vi "ABB configure locked rotor.vi"() -> ()   [LabVIEW 2017]
uses:
  ABB global.vi
panel:
  in  "Exit":bool
  in  "Locked Rotor Test":T1={"Number Values"=8, "Tolerance (%)"=2.0, "Value (% rated) "=[1.15, 1.0, 0.91, 0.78, 0.66, 0.55, 0.42, 0.3], "Hold time (sec)"=2.0}
  # "Configure Locked Rotor Test"
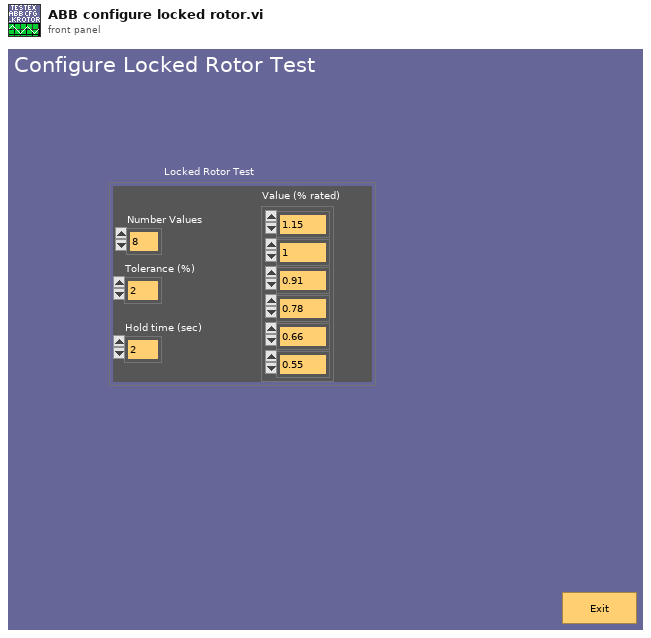
[diagram p1: front panel]
types:
  T1 = cluster{"Number Values":i32, "Tolerance (%)":dbl, "Value (% rated) ":dbl[], "Hold time (sec)":dbl}
  T2 = cluster{"Number Values":i32, "Tolerance":dbl, "Value (ratio) ":dbl[], "Hold time (sec)":dbl}
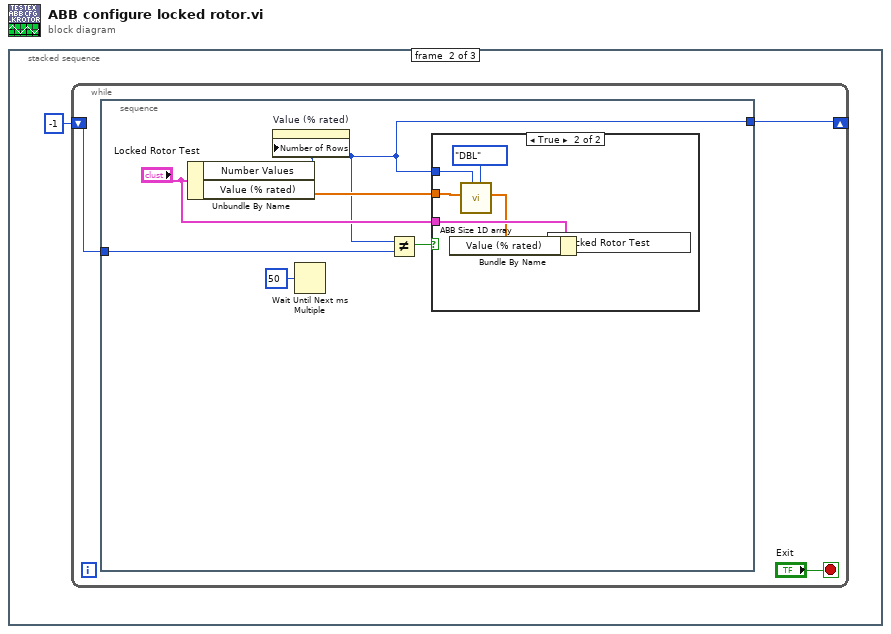
[diagram p0: block diagram]
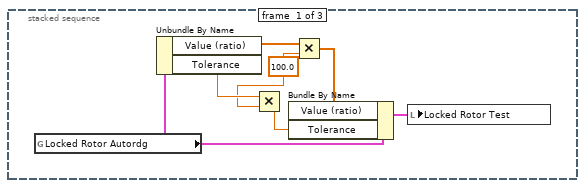
[diagram p2: hidden frame]
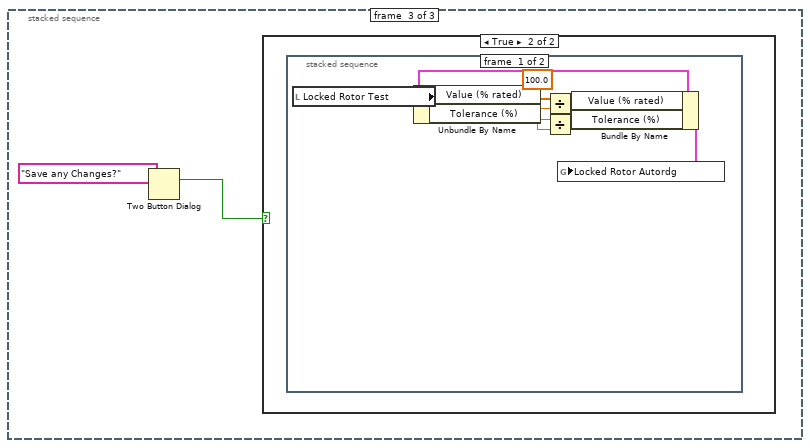
[diagram p4: hidden frame]
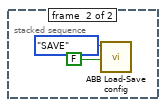
[diagram p6: hidden frame]
diagram:
  n1 = stacked-sequence {
    frame #0 {
      w2 = 100.0
      n2 = global read "ABB global.vi" "Locked Rotor Autordg"() -> (w6:T2)
      n3 = Unbundle By Name(w6) -> ("Value (ratio)"=w7:dbl[], "Tolerance"=w3:dbl)
      n4 = Multiply(x=w3, y=w2) -> (x*y=w1:dbl)
      n5 = Multiply(x=w7, y=w2) -> (x*y=w5:dbl[])
      n6 = Bundle By Name(cluster=w6, "Value (ratio)"=w5, "Tolerance"=w1) -> (w4:T2)
      n7 = local write "Locked Rotor Test"(w4) -> ()
    }
    frame #1 {
      n8 = while {
        shift-right: [w9] -> _
        shift-left: -1 ("Number Values") -> [w10]
        stop <- "Exit" stop-if-true
        n9 = stacked-sequence {
          tunnel: w10 -> [w15]
          tunnel: [w12] -> w9
          frame #0 {
            n10 = Unbundle By Name("Locked Rotor Test") -> ("Number Values"=w12:i32, "Value (% rated)"=w13:dbl[])
            n11 = property on="Value (% rated)" class="Arr (strict)"("Number of Rows"=w12) -> ()  [unwired: 2 in, 2 out]
            n12 = Wait Until Next ms Multiple(millisecond multiple=u32 50) -> ()  [unwired: 1 out]
            n13 = Not Equal?(x=w12, y=w15) -> (x != y?=w14:bool)
            n14 = case shown="True" w14 {
              tunnel: "Locked Rotor Test" -> [_ w23]
              tunnel: w13 -> [_ w21]
              tunnel: w12 -> [_ w19]
              frame False {
              }
              frame True {
                n15 = call "ABB Size 1D array.vi"("Type"=enum16{"Integer", "DBL", "STRING", "BOOLEAN"}."DBL", "Size"=w19, "DBL Array In"=w21) -> ("DBL Array out"=w18:dbl[])  [unwired: 5 in, 3 out]
                n16 = Bundle By Name(cluster=w23, "Value (% rated)"=w18) -> (w22:T1)
                n17 = local write "Locked Rotor Test"(w22) -> ()
              }
            }
          }
        }
      }
    }
    frame #2 {
      n18 = Two Button Dialog(message="Save any Changes?") -> (T button?=w25:bool)  [unwired: 2 in]
      n19 = case shown="True" w25 {
        frame False {
        }
        frame True {
          n20 = stacked-sequence {
            frame #0 {
              w27 = 100.0 ("Numeric")
              n21 = local read "Locked Rotor Test"() -> (w30:T1)
              n22 = Unbundle By Name(w30) -> ("Value (% rated)"=w32:dbl[], "Tolerance (%)"=w26:dbl)
              n23 = Divide(x=w32, y=w27) -> (x/y=w31:dbl[])
              n24 = Divide(x=w26, y=w27) -> (x/y=w28:dbl)
              n25 = Bundle By Name(cluster=w30, "Value (% rated)"=w31, "Tolerance (%)"=w28) -> (w29:T1)
              n26 = global write "ABB global.vi" "Locked Rotor Autordg"(w29) -> ()
            }
            frame #1 {
              n27 = call "ABB Load-Save config.vi"("confirm save"=FALSE, "Mode"=enum16{"LOAD", "SAVE"}."SAVE") -> ()  [unwired: 10 in]
            }
          }
        }
      }
    }
  }
